vi "RS485.vi"(8 "error in":errorcluster, 9 "Endereco":string, 10 "ComPort":refnum<visa-resource-name>) -> (0 "error out":errorcluster)   [LabVIEW 2019]
panel:
  out "Saidas":string[](array[string])
  in  "CRC":string
  in  "DadosRequisicao":string
  in  "Funcao":string
  out "return count":u32
  in  "Enum":enum16{"Abrir", "Fechar", "Medir"}(ring)
  out "Saida":string
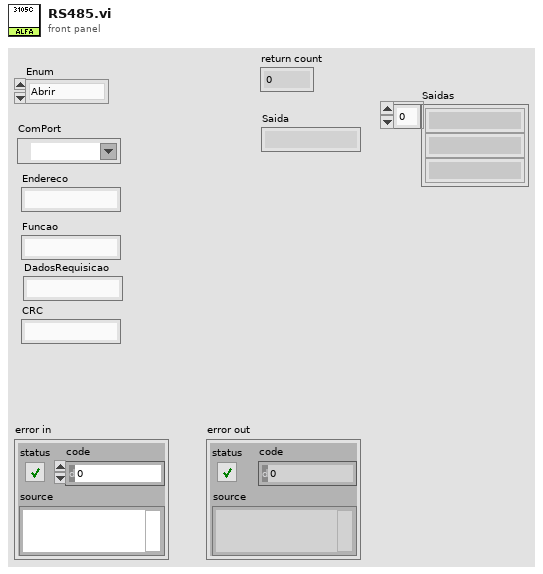
[diagram p1: front panel]
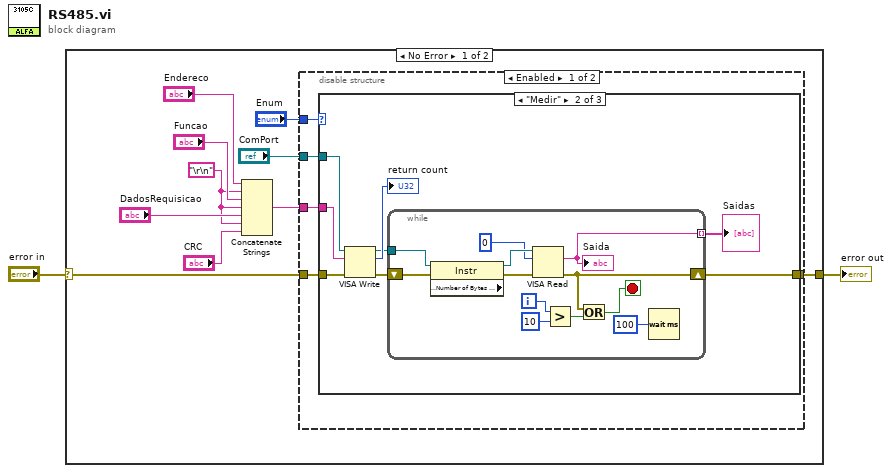
[diagram p0: block diagram]
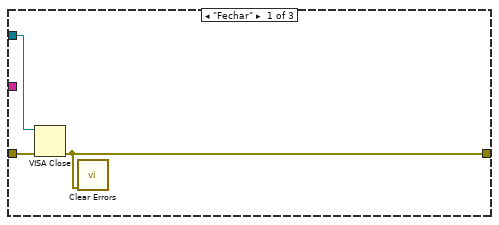
[diagram p2: hidden frame]
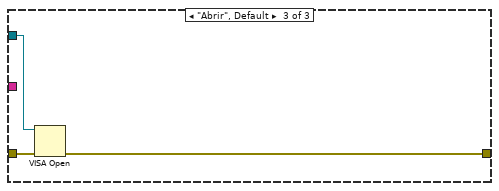
[diagram p3: hidden frame]
diagram:
  n1 = case shown="No Error" "error in" {
    selector: "error in" -> [w11 w44]
    tunnel: [w10 w44] -> w1
    frame No Error {
      w5 = "\r\n"
      n2 = Concatenate Strings("Endereco", w5, "Funcao", w5, "DadosRequisicao", w5, "CRC") -> (w3:string)
      n3 = disable-structure shown="Enabled" {
        disable-tunnel: "ComPort" -> [w17 _]
        disable-tunnel: w11 -> [w16 _]
        disable-tunnel: w3 -> [w15 _]
        disable-tunnel: [w14 _] -> w10
        disable-tunnel: "Enum" -> [w13 _]
        frame Enabled {
          n4 = case shown="\"Medir\"" w13 {
            tunnel: w17 -> [w18 w27 w43]
            tunnel: w16 -> [w19 w28 w42]
            tunnel: w15 -> [_ w24 _]
            tunnel: [w20 w26 w41] -> w14
            frame "Fechar" {
              n5 = VISA Close(VISA resource name=w18, error in (no error)=w19) -> (error out=w20:errorcluster)
              n6 = call <vilib>:"Clear Errors.vi"("error in (no error)"=w20) -> ()  [unwired: 5 in, 2 out]
            }
            frame "Medir" {
              n7 = VISA Write(VISA resource name=w27, write buffer=w24, error in (no error)=w28) -> (VISA resource name out=w22:refnum<visa-resource-name>, return count=→"return count":u32, error out=w23:errorcluster)
              n8 = while {
                tunnel: w22 -> [w39]
                shift-right: [w31] -> w26
                shift-left: w23 -> [w40]
                tunnel: [w35] -> w21 mode=indexing
                i -> [w32]
                stop <- w30 stop-if-true
                n9 = property class="Instr" props=["Serial Settings:Number of Bytes at Serial Port"](reference=w39, error in=w40) -> (reference out=w37:refnum<visa-resource-name>, error out=w38:errorcluster)  [unwired: 1 out]
                n10 = VISA Read(VISA resource name=w37, byte count=0, error in (no error)=w38) -> (read buffer=w35:string, error out=w31:errorcluster)  [unwired: 2 out]
                "Saida" <- w35
                n11 = Greater?(x=w32, y=10) -> (0:w33:bool)
                n12 = Or(x=w31, y=w33) -> (x .or. y?=w30:bool)
                n13 = Wait (ms)(milliseconds to wait=u32 100) -> ()  [unwired: 1 out]
              }
              "Saidas" <- w21
            }
            frame "Abrir", Default {
              n14 = VISA Open(error in (no error)=w42, VISA resource name=w43) -> (error out=w41:errorcluster)  [unwired: 3 in, 1 out]
            }
          }
        }
        frame Disabled {
        }
      }
    }
    frame Error {
    }
  }
  "error out" <- w1
